vi "LX.vi"() -> ()   [LabVIEW 2020]
panel:
  in  "BX":dbl
  in  "LX":dbl
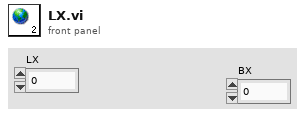
[diagram p1: front panel]
diagram:
